vi "ErrorHandling_GetAllError.vi"(8 "Fehler (Eingang, kein Fehler)":errorcluster caption="Error_In", 11 "Referenz_In":refnum<visa-resource-name>) -> (0 "Fehler (Ausgang)":errorcluster caption="Error_Out", 1 "communication_data":T1, 2 "Error List":cluster{"ErrorCode":i32, "Error":string}[](array[cluster]), 3 "Referenz_Out":refnum<visa-resource-name>)   [LabVIEW 2018, in "OXYGEN.lvlib"]
doc: "Queries all entries the Error Queue"
uses:
  OXYGEN.lvlib
  TypeDefs/Cluster_RawCommData.ctl
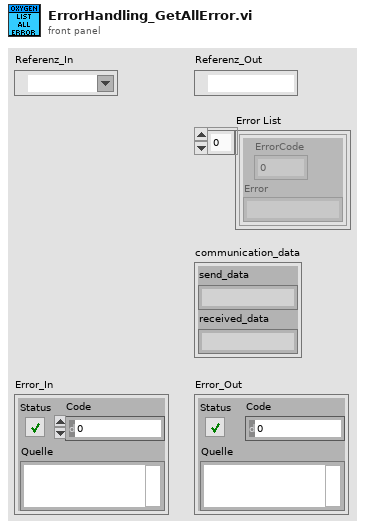
[diagram p1: front panel]
types:
  T1 = typedef "OXYGEN.lvlib/Cluster_RawCommData.ctl" = cluster{"send_data":string, "received_data":string}
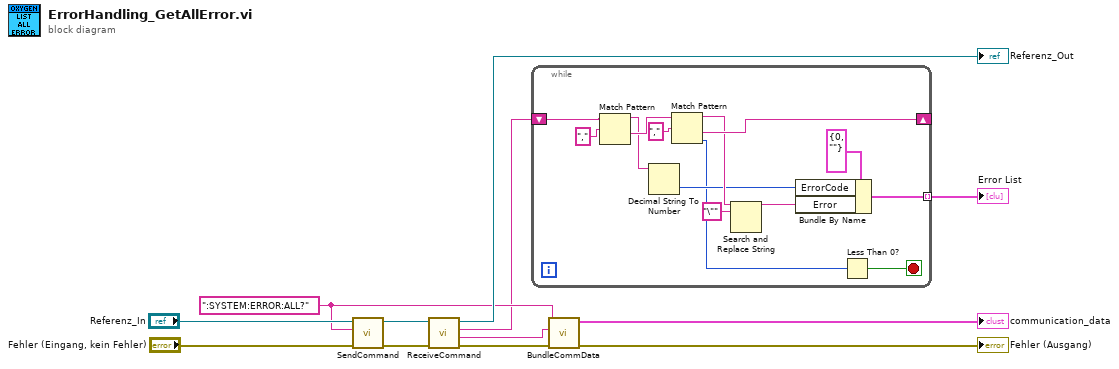
[diagram p0: block diagram]
diagram:
  w6 = ":SYSTEM:ERROR:ALL?" ("Schreibpuffer")
  n1 = call "SendCommand.vi"("error in (no error)"="Fehler (Eingang, kein Fehler)", "String to Send"=w6, "OXY_SCPI Reseource In"="Referenz_In") -> ("error out"=w8:errorcluster, "OXY_SCPI Reseource Out"=w7:refnum<visa-resource-name>)  [unwired: 7 in]
  n2 = call "ReceiveCommand.vi"("error in (no error)"=w8, "OXY_SCPI Reseource In"=w7) -> ("error out"=w4:errorcluster, "received Data with Header"=w5:string, "received Data"=w2:string, "OXY_SCPI Reseource Out"=→"Referenz_Out":refnum<visa-resource-name>)  [unwired: 6 in]
  n3 = while {
    shift-right: [w22] -> _
    shift-left: w2 -> [w23]
    tunnel: [w15] -> w1 mode=indexing
    stop <- w13 stop-if-true
    n4 = Match Pattern(string=w23, regular expression=",") -> (before substring=w17:string, after substring=w26:string)  [unwired: 1 in, 2 out]
    n5 = Decimal String To Number(string=w17) -> (number=w16:i32)  [unwired: 2 in, 1 out]
    n6 = Match Pattern(string=w26, regular expression=",") -> (before substring=w19:string, after substring=w22:string, offset past match=w14:i32)  [unwired: 1 in, 1 out]
    n7 = Search and Replace String(input string=w19, search string="\"") -> (result string=w20:string)  [unwired: 6 in, 3 out]
    n8 = Bundle By Name(cluster=cluster{"ErrorCode":i32, "Error":string} {"ErrorCode"=0, "Error"=""}, "ErrorCode"=w16, "Error"=w20) -> (w15:cluster{"ErrorCode":i32, "Error":string})
    n9 = Less Than 0?(x=w14) -> (x < 0?=w13:bool)
  }
  "Error List" <- w1
  n10 = call "BundleCommData.vi"("error in (no error)"=w4, "received_data"=w5, "send_data"=w6) -> ("error out"=→"Fehler (Ausgang)":errorcluster, "communication_data"=→"communication_data":T1)  [unwired: 7 in]
